vi "SPI_Open_Device_By_Name_LocID.vi"(2 "LocID":u32, 3 "DeviceName":string) -> (0 "Handle":u32, 1 "FTC_Status":u32)   [LabVIEW 2010]
uses:
  FTCSPI.dll
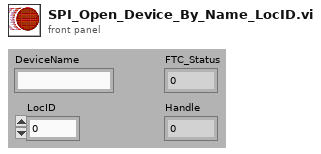
[diagram p1: front panel]
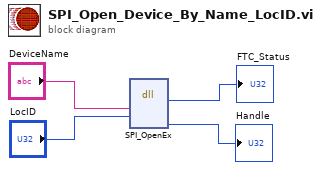
[diagram p0: block diagram]
diagram:
  n1 = dll-call lib="C:/Users/Administrator/Documents/GitHub/labview/FPGA/FTCSPI.dll" fn="SPI_OpenEx"("DeviceName"="DeviceName", "LocID"="LocID") -> ("FTC_Status"=→"FTC_Status":u32, "Handle"=→"Handle":u32)  [unwired: 6 in, 2 out]
